vi "Framework.Get All Transfers.vi"(11 "Framework in":refnum<class "Framework.lvclass">) -> (2 "All Transfers":refnum<class "Transfer.lvclass">[](array[class]), 3 "Framework out":refnum<class "Framework.lvclass">)   [LabVIEW 2017, in "DSF Core.lvlib" / "Framework.lvclass"]
uses:
  Framework.lvclass
  Transfer/Transfer.lvclass
  Framework.lvclass/Framework.ctl
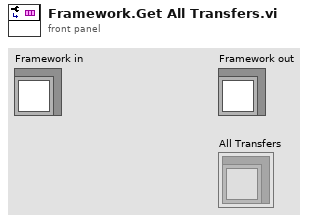
[diagram p1: front panel]
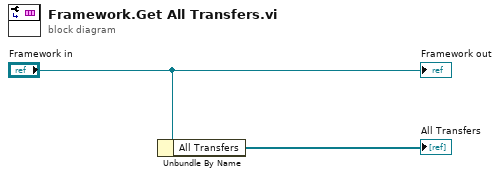
[diagram p0: block diagram]
diagram:
  n1 = Unbundle By Name("Framework in") -> ("All Transfers"=→"All Transfers":refnum<class "Transfer.lvclass">[])
  "Framework out" <- "Framework in"
